vi "三角波发生器.vi"() -> ()   [LabVIEW 2014]
uses:
  <vilib>/Waveform/DWDTOps.llb/Digital Pattern Generator (Ramp).vi
panel:
  in  "旋钮":i32(knob) scale=0.0..10.0
  out "波形图表":dynamicdata(graph)
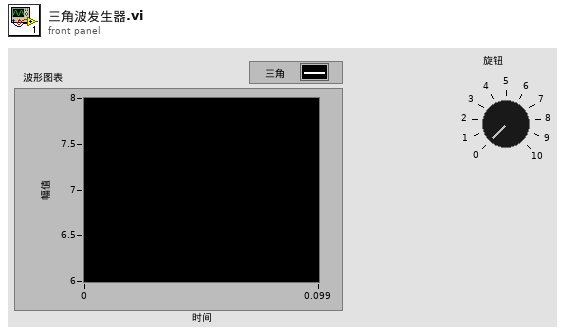
[diagram p1: front panel]
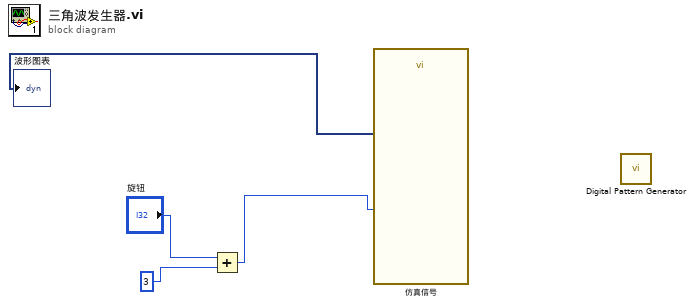
[diagram p0: block diagram]
diagram:
  n1 = Add(x="旋钮", y=3) -> (x+y=w1:i32)
  n2 = call "仿真信号"("Offset"=w1) -> ("三角"=→"波形图表":dynamicdata)  [unwired: 13 in, 1 out]
  n3 = call-poly <vilib>:"Digital Pattern Generator.vi"() -> ()  [unwired: 10 in, 2 out]
